vi "Check Calibration Validity.vi"(0 "RFPM Handle In":refnum<k15>, 5 "Calibration Interval Check":T1={"Check Calibration Interval?"=FALSE, "Temperature Interval (deg C)"=0.0, "Calibration Interval (days)"=0.0, "Out of Calibration Message"=enum."Error"} {"Calibration Interval (days)" format="%#_13g"; "Temperature Interval (deg C)" format="%#_13g"}, 11 "error in":errorcluster) -> (4 "RFPM Handle Out":refnum<k15>, 15 "error out":errorcluster)   [LabVIEW 2023, in "RFFixtureCharact.RFPM.lvlib" / "RF Subsystem Session Provider.lvclass"]
uses:
  RF Subsystem Session Provider.lvclass
  Controls/Calibration Check.ctl
  <vilib>/Utility/error.llb/Error Cluster From Error Code.vi
  <instrlib>/niRFPM/niRFPM.llb/NI-RFPM Read Available User Vector Calibration Information.vi
  <instrlib>/niRFPM/niRFPM.llb/NI-RFPM Read Available User Source Offset Calibration Information.vi
  <instrlib>/niRFPM/niRFPM.llb/NI-RFPM Read Available User Receiver Offset Calibration Information.vi
  <vilib>/ErrorRing/Error Ring.xnode
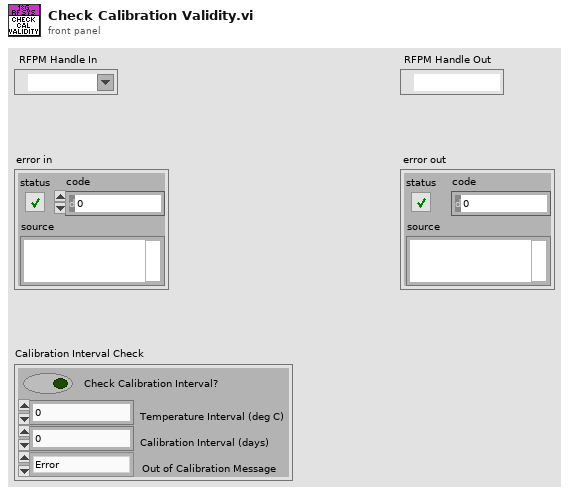
[diagram p1: front panel]
types:
  T1 = typedef "RFFixtureCharact.RFPM.lvlib/RF Subsystem Session Provider.lvclass/Calibration Check.ctl" = cluster{"Check Calibration Interval?":bool, "Temperature Interval (deg C)":dbl, "Calibration Interval (days)":dbl, "Out of Calibration Message":enum16{"Warning", "Error"}}
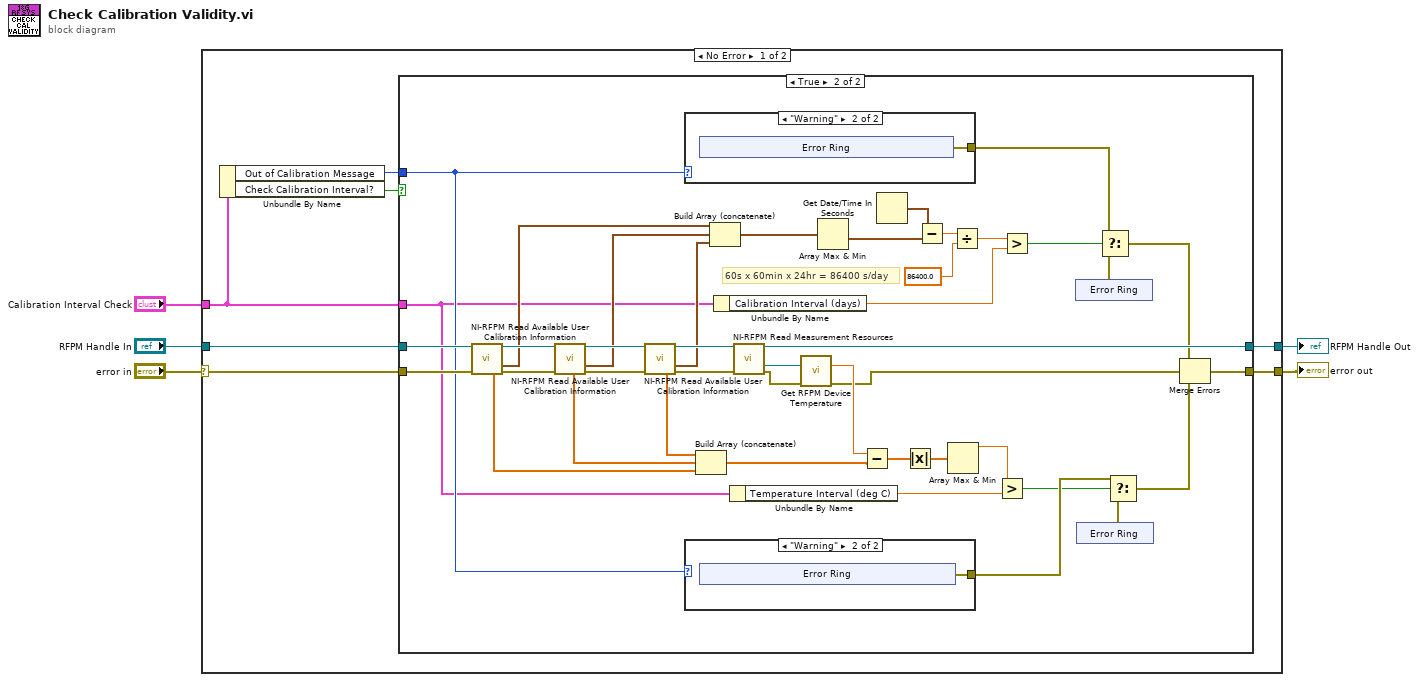
[diagram p0: block diagram]
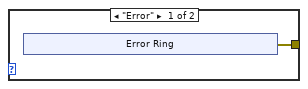
[diagram p3: hidden frame]
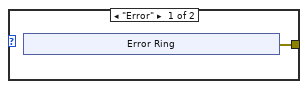
[diagram p4: hidden frame]
diagram:
  n1 = case shown="No Error" "error in" {
    selector: "error in" -> [w6 w83]
    tunnel: [w12 w84] -> w5
    tunnel: "RFPM Handle In" -> [w11 w84]
    tunnel: [w10 w83] -> w3
    tunnel: "Calibration Interval Check" -> [w7 _]
    frame No Error {
      n2 = Unbundle By Name(w7) -> ("Out of Calibration Message"=w8:enum16{"Warning", "Error"}, "Check Calibration Interval?"=w9:bool)
      n3 = case shown="True" w9 {
        tunnel: [w14 w46] -> w12
        tunnel: w11 -> [w14 w45]
        tunnel: w6 -> [w13 w44]
        tunnel: [w13 w22] -> w10
        tunnel: w7 -> [_ w19]
        tunnel: w8 -> [_ w20]
        frame False {
        }
        frame True {
          # "60s x 60min x 24hr = 86400 s/day"
          n4 = call-poly <instrlib>:"NI-RFPM Read Available User Calibration Information.vi"("instrument handle in"=w45, "error in"=w44) -> ("instrument handle out"=w42:refnum<k15>, "Dates\\Times"=w35:timestamp[], "Temperatures"=w37:dbl[], "error out"=w43:errorcluster)  [unwired: 8 in, 2 out]
          n5 = call-poly <instrlib>:"NI-RFPM Read Available User Calibration Information.vi"("instrument handle in"=w42, "error in"=w43) -> ("instrument handle out"=w41:refnum<k15>, "Dates\\Times"=w34:timestamp[], "Temperatures"=w38:dbl[], "error out"=w40:errorcluster)  [unwired: 8 in, 2 out]
          n6 = call-poly <instrlib>:"NI-RFPM Read Available User Calibration Information.vi"("instrument handle in"=w41, "error in"=w40) -> ("instrument handle out"=w51:refnum<k15>, "Dates\\Times"=w33:timestamp[], "Temperatures"=w39:dbl[], "error out"=w50:errorcluster)  [unwired: 8 in, 2 out]
          n7 = case shown="\"Warning\"" w20 {
            tunnel: [w58 w64] -> w30
            frame "Error" {
              n8 = xnode "Error Ring"() -> ("error out"=w58:errorcluster)
            }
            frame "Warning" {
              n9 = xnode "Error Ring"() -> ("error out"=w64:errorcluster)
            }
          }
          n10 = case shown="\"Warning\"" w20 {
            tunnel: [w70 w76] -> w27
            frame "Error" {
              n11 = xnode "Error Ring"() -> ("error out"=w70:errorcluster)
            }
            frame "Warning" {
              n12 = xnode "Error Ring"() -> ("error out"=w76:errorcluster)
            }
          }
          n13 = Build Array (concatenate)(w39, w38, w37) -> (w36:dbl[])
          n14 = Build Array (concatenate)(w35, w34, w33) -> (w32:timestamp[])
          n15 = Unbundle By Name(w19) -> ("Calibration Interval (days)"=w31:dbl)
          n16 = Unbundle By Name(w19) -> ("Temperature Interval (deg C)"=w21:dbl)
          n17 = call <instrlib>:"NI-RFPM Read Measurement Resources.vi"("NI-5530 handle in"=w51, "error in"=w50) -> ("NI-5530 handle out"=w46:refnum<k15>, "Switch handle"=w18:refnum<k15>, "error out"=w17:errorcluster)  [unwired: 9 in, 2 out]
          n18 = call "Get RFPM Device Temperature.vi"("IVISwitch Handle in"=w18, "error in"=w17) -> ("Device Temperature"=w16:dbl, "error out"=w15:errorcluster)  [unwired: 11 in, 1 out]
          n19 = Array Max & Min(array=w32) -> (min value=w52:timestamp)  [unwired: 3 out]
          n20 = Subtract(x=w16, y=w36) -> (x-y=w49:dbl[])
          n21 = Get Date/Time In Seconds() -> (seconds since 1Jan1904=w53:timestamp)
          n22 = Absolute Value(x=w49) -> (abs(x)=w48:dbl[])
          n23 = Subtract(x=w53, y=w52) -> (x-y=w54:dbl)
          n24 = Array Max & Min(array=w48) -> (max value=w47:dbl)  [unwired: 3 out]
          n25 = Divide(x=w54, y=86400.0) -> (x/y=w55:dbl)
          n26 = Greater?(x=w47, y=w21) -> (0:w25:bool)
          n27 = Greater?(x=w55, y=w31) -> (0:w28:bool)
          n28 = xnode "Error Ring"() -> ("error out"=w29:errorcluster)
          n29 = xnode "Error Ring"() -> ("error out"=w26:errorcluster)
          n30 = Select(t=w30, s=w28, f=w29) -> (s? t:f=w24:errorcluster)
          n31 = Select(t=w27, s=w25, f=w26) -> (s? t:f=w23:errorcluster)
          n32 = Merge Errors(w24, w15, w23) -> (w22:errorcluster)
        }
      }
    }
    frame Error {
    }
  }
  "RFPM Handle Out" <- w5
  "error out" <- w3
